vi "get Norm by id.vi"(8 "error in (no error)":errorcluster caption="Fehler (Eingang, kein Fehler)", 10 "id":i32, 11 "Report (Eingang)":refnum<class "Report.lvclass">) -> (0 "error out":errorcluster caption="Fehler (Ausgang)", 1 "id found":bool, 2 "Norm.lvclass":refnum<class "Norm.lvclass">, 3 "Report (Ausgang)":refnum<class "Report.lvclass">, 4 "index":i32)   [LabVIEW 2013, in "DatenKlassen.lvlib" / "Report.lvclass"]
doc: "Ein Norm-Objekt finden anhand einer ID"
uses:
  Report.lvclass
  Norm/Norm.lvclass
  Report.lvclass/Report.ctl
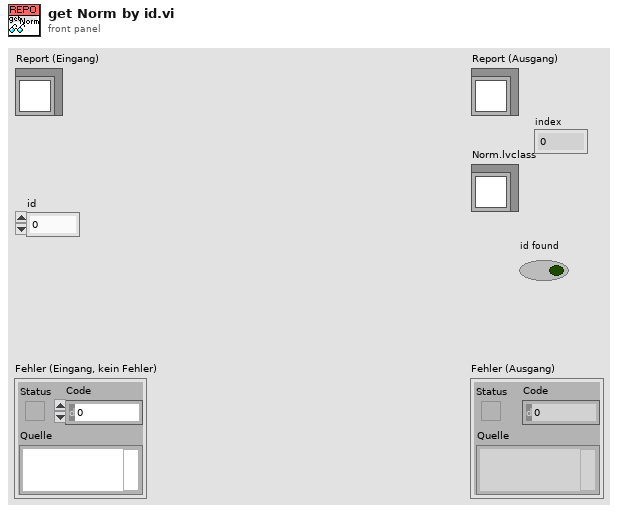
[diagram p1: front panel]
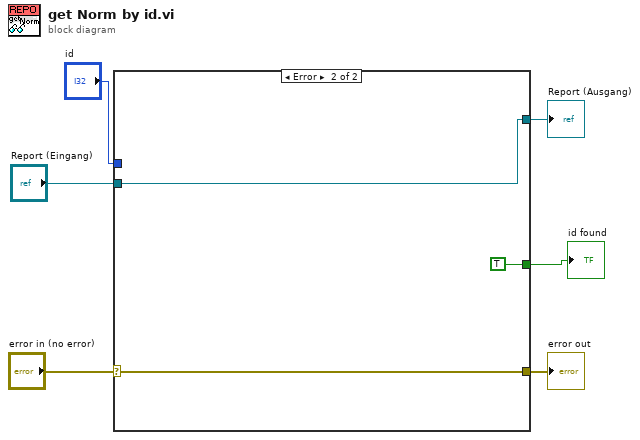
[diagram p0: block diagram]
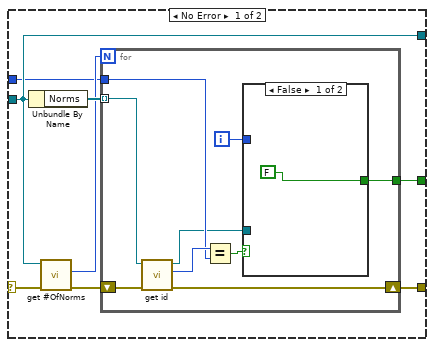
[diagram p2: hidden frame]
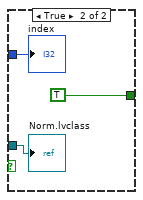
[diagram p3: hidden frame]
diagram:
  n1 = case shown="Error" "error in (no error)" {
    selector: "error in (no error)" -> [w11 w29]
    tunnel: [w9 w29] -> w5
    tunnel: [w13 w30] -> w3
    tunnel: "Report (Eingang)" -> [w13 w30]
    tunnel: "id" -> [w8 _]
    tunnel: [w7 TRUE ("id found")] -> w1
    frame No Error {
      n2 = Unbundle By Name(w13) -> ("Norms"=w14:refnum<class "Norm.lvclass">[])
      n3 = call-dynamic "get #OfNorms.vi"("error in (no error)"=w11, "Report (Eingang)"=w13) -> ("error out"=w10:errorcluster, "#OfTests"=w12:u32)  [unwired: 7 in, 1 out]
      n4 = for {
        N: w12 -> [_]
        tunnel: w14 -> [w23] mode=indexing
        shift-right: [w21] -> w9
        shift-left: w10 -> [w22]
        tunnel: w8 -> [w19]
        tunnel: [w15] -> w7
        i -> [w16]
        n5 = call-dynamic "get id.vi"("error in (no error)"=w22, "Norm (Eingang)"=w23) -> ("error out"=w21:errorcluster, "id"=w20:i32, "Norm (Ausgang)"=w17:refnum<class "Norm.lvclass">)  [unwired: 7 in]
        n6 = Equal?(x=w20, y=w19) -> (x = y?=w18:bool)
        n7 = case shown="False" w18 {
          tunnel: w17 -> [_ w27]
          tunnel: w16 -> [_ w26]
          tunnel: [FALSE ("id found") TRUE] -> w15
          frame False {
          }
          frame True {
            "Norm.lvclass" <- w27
            "index" <- w26
          }
        }
      }
    }
    frame Error {
    }
  }
  "error out" <- w5
  "Report (Ausgang)" <- w3
  "id found" <- w1
